vi "MICSD Format Hex Table.vi"(3 "Columns":u8=16, 4 "Read Data":u8[](array[numeric]), 5 "Start Address":u8 format="%04x") -> (1 "String":string)   [LabVIEW 2020]
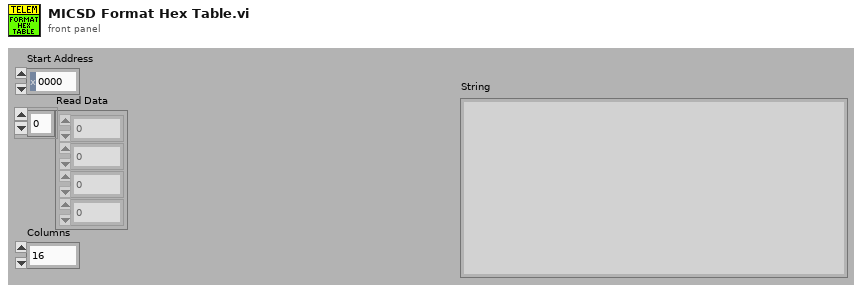
[diagram p1: front panel]
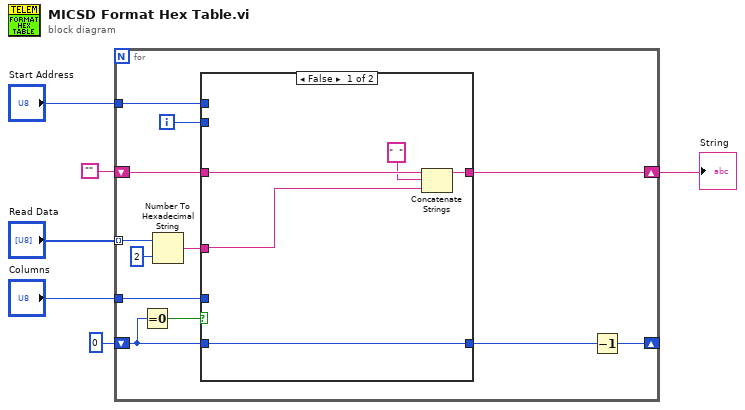
[diagram p0: block diagram]
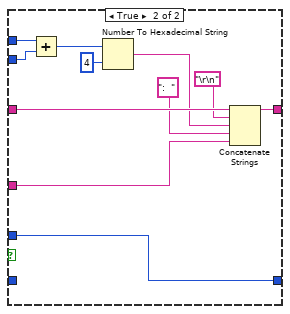
[diagram p2: hidden frame]
diagram:
  n1 = for {
    tunnel: "Read Data" -> [w13] mode=indexing
    shift-right: [w18] -> _
    shift-left: u8 0 ("Columns") -> [w17]
    tunnel: "Columns" -> [w10]
    shift-right: [w8] -> w2
    shift-left: "" -> [w9]
    tunnel: "Start Address" -> [w7]
    i -> [w11]
    n2 = Equal To 0?(x=w17) -> (x = 0?=w16:bool)
    n3 = Number To Hexadecimal String(1:i16 2 ("width (-)"), 2:w13) -> (0:w12:string)
    n4 = case shown="False" w16 {
      tunnel: w17 -> [w23 _]
      tunnel: w10 -> [_ w33]
      tunnel: [w23 w33] -> w15
      tunnel: w12 -> [w19 w28]
      tunnel: w11 -> [_ w25]
      tunnel: w9 -> [w22 w32]
      tunnel: [w21 w27] -> w8
      tunnel: w7 -> [_ w26]
      frame False {
        n5 = Concatenate Strings(w22, "  ", w19) -> (w21:string)
      }
      frame True {
        n6 = Add(x=w26, y=w25) -> (x+y=w24:i32)
        n7 = Number To Hexadecimal String(1:i16 4 ("width (-)"), 2:w24) -> (0:w30:string)
        n8 = Concatenate Strings(w32, "\r\n", w30, ":  ", w28) -> (w27:string)
      }
    }
    n9 = Decrement(x=w15) -> (x-1=w18:u8)
  }
  "String" <- w2
